vi "DirtyHighPass(SubVI).vi"(6 "Enable":bool, 8 "tau":dbl, 10 "dt[s]":dbl, 11 "Numeric in":dbl) -> (3 "Numeric out":dbl)   [LabVIEW 2017]
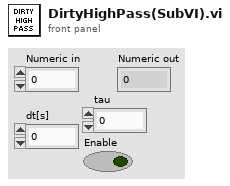
[diagram p1: front panel]
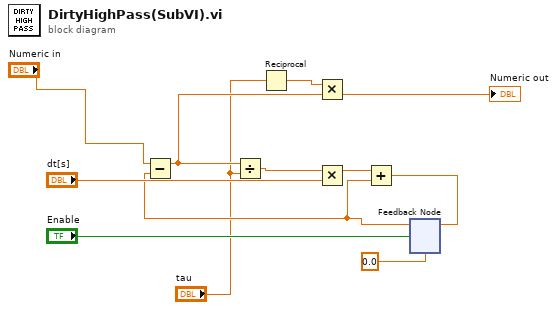
[diagram p0: block diagram]
diagram:
  n1 = Reciprocal(x="tau") -> (1/x=w2:dbl)
  n2 = feedback #1(0.0) -> (w8:dbl)
  n3 = Subtract(x="Numeric in", y=w8) -> (x-y=w7:dbl)
  n4 = Divide(x=w7, y="tau") -> (x/y=w12:dbl)
  n5 = Multiply(x=w2, y=w7) -> (x*y=→"Numeric out":dbl)
  n6 = Multiply(x=w12, y="dt[s]") -> (x*y=w11:dbl)
  n7 = Add(x=w11, y=w8) -> (x+y=w9:dbl)
  n8 = feedback-in #1(w9, "Enable") -> ()
